vi "WT210 IEC 2015 Setup.vi"(0 "VISA Input":refnum<visa-resource-name>, 5 "V Range (6: 600V)":u16(ring)=4 items=["Auto", "15V", "30V", "60V", "150V", "300V", "600V"], 7 "A Range (12: 20A)":u16(ring)=10 items=["Auto", "5mA", "10mA", "20mA", "50mA", "100mA", "200mA", "0.5A", "1A", "2A", "5A", "10A", "20A", "50mV", "100mV", "200mV", "2.5V", "5V", "10V"], 9 "Sample Rate (1: 0.25s)":u16(ring)=1 items=["0.1s", "0.25s", "0.5s", "1s", "2s", "5s"], 11 "error in (no error)":errorcluster) -> (2 "VTHD":sgl format="%.3g", 4 "VISA Output":refnum<visa-resource-name>, 6 "Header File":string[][](array[string]), 15 "error out":errorcluster)   [LabVIEW 2018]
uses:
  <vilib>/Utility/error.llb/whitespace.ctl
  Yokogawa WT200 Series.lvlib
panel:
  in  "Tab Control":enum32{"Main", "Debug"}(tab)
  out "Sample Rate":string
  out "V Range":string
  out "A Range":string
  out "Instrument ID":string
  out "Date & Time":string
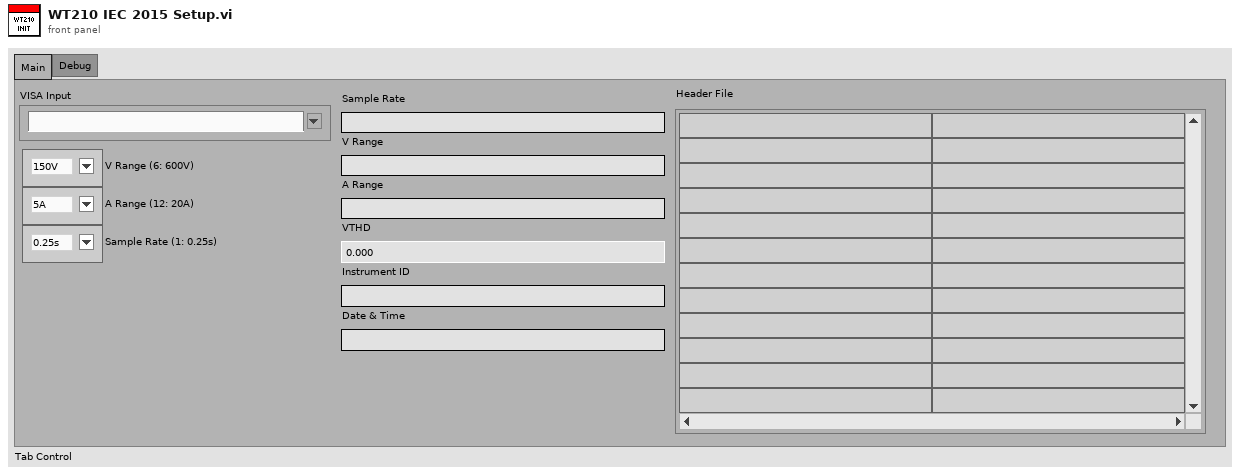
[diagram p1: front panel]
types:
  T1 = typedef "whitespace.ctl" = u16
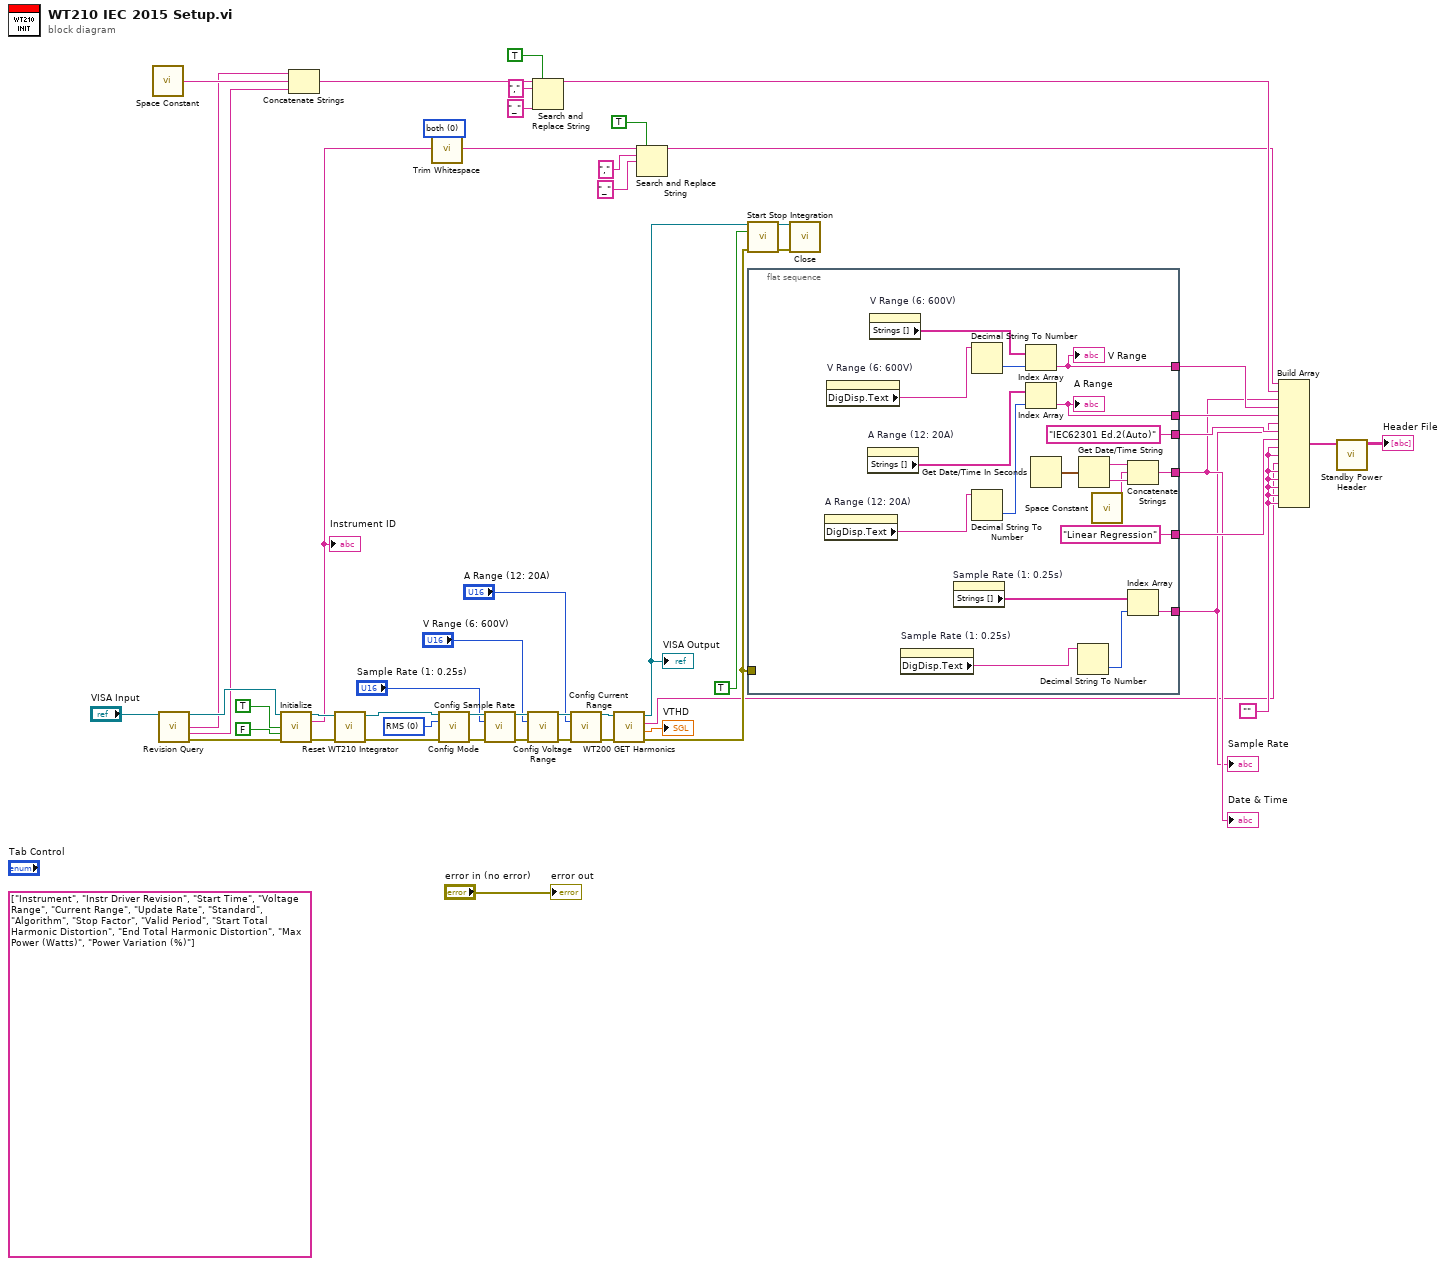
[diagram p0: block diagram]
diagram:
  w20 = T1 0 items=["both", "start of string", "end of string"] ("location (both)")
  w33 = ""
  (unwired) string[] ["Instrument", "Instr Driver Revision", "Start Time", "Voltage Range", "Current Range", "Update Rate", "Standard", "Algorithm", "Stop Factor", "Valid Period", "Start Total Harmonic Distortion", "End Total Harmonic Distortion", "Max Power (Watts)", "Power Variation (%)"]
  w45 = u16 0 items=["RMS", "V-MEAN", "DC"] ("Mode (0: RMS)")
  n1 = call <vilib>:"Space Constant.vi"() -> ("String"=w36:string)
  n2 = call "Revision Query.vi"("VISA resource name"="VISA Input") -> ("VISA resource name out"=w47:refnum<visa-resource-name>, "Instr Driver Revision"=w35:string, "Instr Firmware Revision"=w34:string, "error out"=w46:errorcluster)  [unwired: 11 in]
  n3 = call "Initialize.vi"("VISA resource name"=w47, "ID Query (T: Check)"=TRUE, "Reset (T: Reset)"=FALSE, "error in (no error)"=w46) -> ("VISA resource name out"=w23:refnum<visa-resource-name>, "Instrument ID"=w21:string, "error out"=w25:errorcluster)  [unwired: 9 in]
  "Instrument ID" <- w21
  n4 = Concatenate Strings(w35, w36, w34) -> (w7:string)
  n5 = call "Reset WT210 Integrator.vi"("error in (no error)"=w25, "VISA resource name"=w23) -> ("error out"=w24:errorcluster, "VISA resource name out"=w22:refnum<visa-resource-name>)  [unwired: 8 in]
  n6 = call <vilib>:"Trim Whitespace.vi"("string"=w21, "location (both)"=w20) -> ("trimmed string"=w2:string)
  n7 = call "Config Mode.vi"("VISA resource name"=w22, "Mode (0: RMS)"=w45, "error in (no error)"=w24) -> ("VISA resource name out"=w43:refnum<visa-resource-name>, "error out"=w44:errorcluster)  [unwired: 11 in]
  n8 = call "Config Sample Rate.vi"("VISA resource name"=w43, "Sample Rate (1: 0.25s)"="Sample Rate (1: 0.25s)", "error in (no error)"=w44) -> ("VISA resource name out"=w51:refnum<visa-resource-name>, "error out"=w53:errorcluster)  [unwired: 11 in]
  n9 = call "Config Voltage Range.vi"("VISA resource name"=w51, "V Range (6: 600V)"="V Range (6: 600V)", "error in (no error)"=w53) -> ("VISA resource name out"=w50:refnum<visa-resource-name>, "error out"=w52:errorcluster)  [unwired: 11 in]
  n10 = Search and Replace String(replace all?=TRUE ("replace all? (F)"), input string=w7, search string=",", replace string="_" ("replace string (\"\")")) -> (result string=w6:string)  [unwired: 4 in, 3 out]
  n11 = call "Config Current Range.vi"("VISA resource name"=w50, "A Range (12: 20A)"="A Range (12: 20A)", "error in (no error)"=w52) -> ("VISA resource name out"=w17:refnum<visa-resource-name>, "error out"=w16:errorcluster)  [unwired: 11 in]
  n12 = call "WT200 GET Harmonics.vi"("error in (no error)"=w16, "VISA Refnum in"=w17) -> ("error out"=w18:errorcluster, "VTHD"=→"VTHD":dbl, "Final Harmonic Content U1"=w14:string, "VISA Refnum out"=w19:refnum<visa-resource-name>)  [unwired: 6 in]
  "VISA Output" <- w19
  n13 = Search and Replace String(replace all?=TRUE ("replace all? (F)"), input string=w2, search string=",", replace string="_" ("replace string (\"\")")) -> (result string=w1:string)  [unwired: 4 in, 3 out]
  n14 = call "Start Stop Integration.vi"("VISA resource name"=w19, "Start/Stop (F: Stop)"=TRUE, "error in (no error)"=w18) -> ("VISA resource name out"=w27:refnum<visa-resource-name>, "error out"=w26:errorcluster)  [unwired: 11 in]
  n15 = flat-sequence {
    tunnel: [w66] -> w42
    tunnel: [w65] -> w41
    tunnel: ["IEC62301 Ed.2(Auto)" ("element")] -> w40
    tunnel: ["Linear Regression" ("element")] -> w39
    tunnel: w18 -> [_]
    tunnel: [w58] -> w32
    tunnel: [w54] -> w31
    frame #0 {
      n16 = property on="A Range (12: 20A)" class="Ring (strict)"() -> ("DigDisp.Text"=w69:string)  [unwired: 2 in, 2 out]
      n17 = property on="V Range (6: 600V)" class="Ring (strict)"() -> ("DigDisp.Text"=w72:string)  [unwired: 2 in, 2 out]
      n18 = property on="A Range (12: 20A)" class="Ring (strict)"() -> ("Strings []"=w67:string[])  [unwired: 2 in, 2 out]
      n19 = property on="V Range (6: 600V)" class="Ring (strict)"() -> ("Strings []"=w70:string[])  [unwired: 2 in, 2 out]
      n20 = property on="Sample Rate (1: 0.25s)" class="Ring (strict)"() -> ("DigDisp.Text"=w55:string)  [unwired: 2 in, 2 out]
      n21 = property on="Sample Rate (1: 0.25s)" class="Ring (strict)"() -> ("Strings []"=w56:string[])  [unwired: 2 in, 2 out]
      n22 = Decimal String To Number(string=w72) -> (number=w71:i32)  [unwired: 2 in, 1 out]
      n23 = Decimal String To Number(string=w69) -> (number=w68:i32)  [unwired: 2 in, 1 out]
      n24 = Index Array(array=w70, index=w71) -> (element=w66:string)
      "V Range" <- w66
      n25 = Index Array(array=w67, index=w68) -> (element=w65:string)
      "A Range" <- w65
      n26 = Get Date/Time In Seconds() -> (seconds since 1Jan1904=w59:timestamp)
      n27 = Decimal String To Number(string=w55) -> (number=w57:i32)  [unwired: 2 in, 1 out]
      n28 = Get Date/Time String(seconds (now)=w59) -> (date string=w61:string, time string=w62:string)  [unwired: 2 in]
      n29 = call <vilib>:"Space Constant.vi"() -> ("String"=w60:string)
      n30 = Concatenate Strings(w61, w60, w62) -> (w58:string)
      n31 = Index Array(array=w56, index=w57) -> (element=w54:string)
    }
  }
  n32 = call "Close.vi"("VISA resource name"=w27, "error in (no error)"=w26) -> ()  [unwired: 13 in, 1 out]
  n33 = Build Array(w1, w6, w32, w42, w41, w31, w40, w39, w33, w33, w14, w33, w33, w33, w33, w33) -> (w12:string[])
  n34 = call "Standby Power Header.vi"("Array"=w12) -> ("Header File"=→"Header File":string[][])  [unwired: 9 in, 1 out]
  "error out" <- "error in (no error)"
  "Sample Rate" <- w31
  "Date & Time" <- w32
